vi "Histerisis.vi"() -> ()   [LabVIEW 2020]
panel:
  out "Boolean 2":bool
  out "Waveform Chart 2":dbl(graph)
  out "Waveform Chart":dbl(graph)
  in  "stop":bool
  in  "x":dbl
  in  "MAX":dbl
  in  "MIN":dbl
  out "Histerísis":bool
  out "Boolean":bool
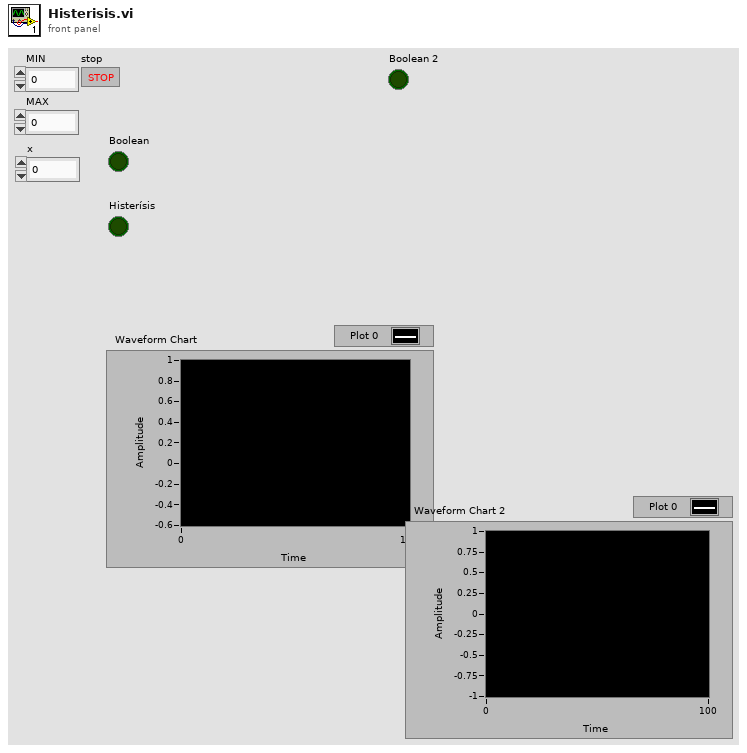
[diagram p1: front panel]
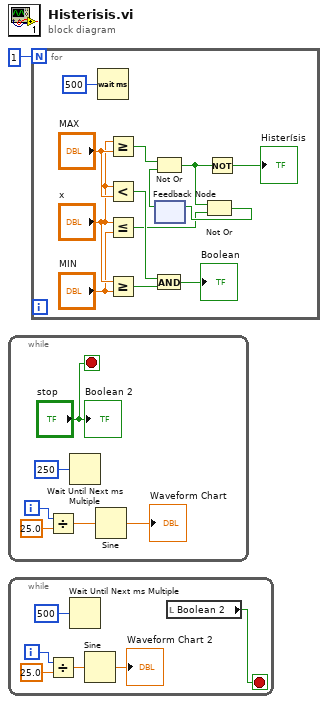
[diagram p0: block diagram]
diagram:
  n1 = while {
    i -> [w6]
    stop <- "stop" stop-if-true
    n2 = Divide(x=w6, y=25.0) -> (x/y=w4:dbl)
    n3 = Wait Until Next ms Multiple(millisecond multiple=u32 250) -> ()  [unwired: 1 out]
    n4 = Sine(x=w4) -> (sin(x)=→"Waveform Chart":dbl)
    "Boolean 2" <- "stop"
  }
  n5 = while {
    i -> [w12]
    stop <- w8 stop-if-true
    n6 = Divide(x=w12, y=25.0) -> (x/y=w10:dbl)
    n7 = Wait Until Next ms Multiple(millisecond multiple=u32 500) -> ()  [unwired: 1 out]
    n8 = Sine(x=w10) -> (sin(x)=→"Waveform Chart 2":dbl)
    n9 = local read "Boolean 2"() -> (w8:bool)
  }
  n10 = for {
    N: 1 -> [_]
    n11 = Wait (ms)(milliseconds to wait=u32 500) -> ()  [unwired: 1 out]
    n12 = Greater Or Equal?(x="x", y="MAX") -> (x >= y?=w19:bool)
    n13 = Less?(x="x", y="MAX") -> (x < y?=w25:bool)
    n14 = Less Or Equal?(x="x", y="MIN") -> (x <= y?=w16:bool)
    n15 = Greater Or Equal?(x="x", y="MIN") -> (x >= y?=w22:bool)
    n16 = And(x=w25, y=w22) -> (x .and. y?=→"Boolean":bool)
    n17 = feedback #1() -> (w17:bool)  [unwired: 1 in]
    n18 = Not Or(1:w17, 2:w19) -> (0:w14:bool)
    n19 = Not Or(1:w16, 2:w14) -> (0:w18:bool)
    n20 = feedback-in #1(w18) -> ()
    n21 = Not(x=w14) -> (.not. x?=→"Histerísis":bool)
  }
